vi "HW1.vi"() -> ()   [LabVIEW 2011]
panel:
  out "positive number":dbl
  out "RUNS":i32
  out "RANDOM VALUE CHART":dbl(graph)
  out "RANDOM VALUES\n         (-1 TO 1)":dbl
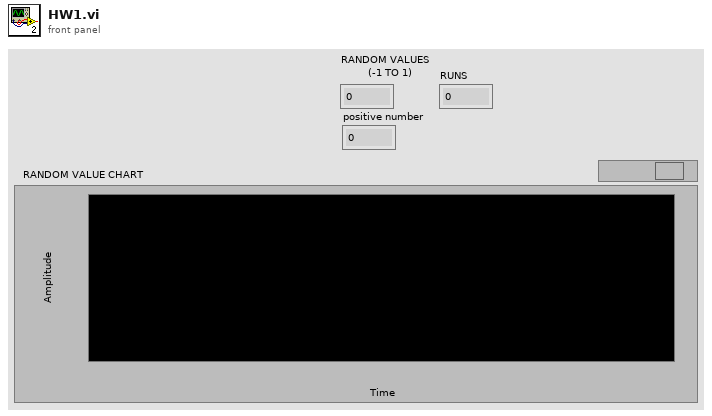
[diagram p1: front panel]
types:
  T1 = enum16{"open", "replace", "create", "open or create", "replace or create", "replace or create with confirmation"}
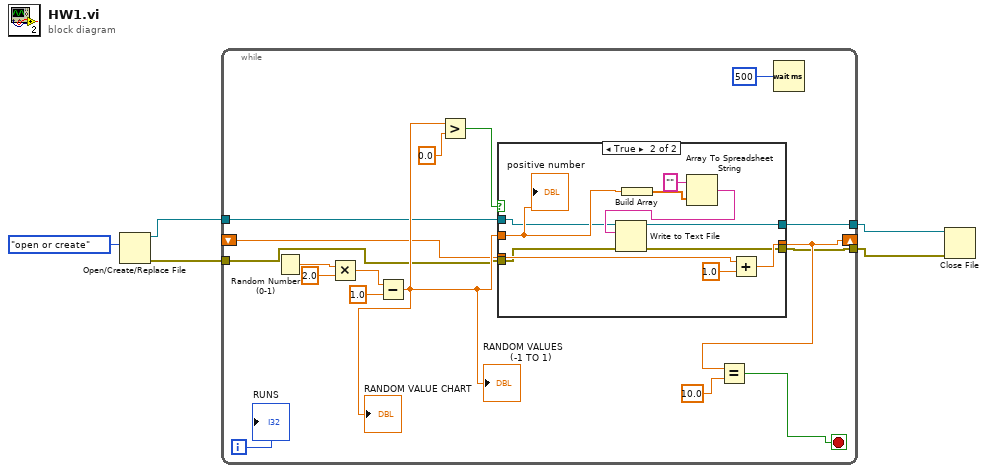
[diagram p0: block diagram]
diagram:
  n1 = Open/Create/Replace File(operation (0:open)=T1."open or create") -> (refnum out=w5:refnum<file>, error out=w3:errorcluster)  [unwired: 5 in, 1 out]
  n2 = while {
    shift-right: [w12] -> _
    shift-left: _ -> [w13]
    tunnel: w5 -> [w9]
    tunnel: [w8] -> w4
    tunnel: w3 -> [w7]
    tunnel: [w6] -> w2
    i -> [w18]
    stop <- w10 stop-if-true
    n3 = Random Number (0-1)() -> (number: 0 to 1=w15:dbl)
    n4 = Multiply(x=w15, y=2.0) -> (x*y=w21:dbl)
    n5 = Subtract(x=w21, y=1.0) -> (x-y=w14:dbl)
    "RANDOM VALUES\n         (-1 TO 1)" <- w14
    "RANDOM VALUE CHART" <- w14
    n6 = Greater?(x=w14, y=0.0) -> (0:w16:bool)
    n7 = case shown="True" w16 {
      tunnel: w14 -> [_ w33]
      tunnel: [w25 w35] -> w12
      tunnel: w13 -> [w25 w34]
      tunnel: w9 -> [w24 w30]
      tunnel: [w24 w29] -> w8
      tunnel: w7 -> [w23 w27]
      tunnel: [w23 w26] -> w6
      frame False {
      }
      frame True {
        n8 = Build Array(w33) -> (w32:dbl[])
        n9 = Array To Spreadsheet String(array=w32, 3:"" ("format string")) -> (spreadsheet string=w31:string)  [unwired: 1 in]
        n10 = Write to Text File(file (use dialog)=w30, text=w31, error in=w27) -> (refnum out=w29:refnum<file>, error out=w26:errorcluster)  [unwired: 1 in, 1 out]
        n11 = Add(x=w34, y=1.0) -> (x+y=w35:dbl)
        "positive number" <- w33
      }
    }
    n12 = Equal?(x=w12, y=10.0) -> (x = y?=w10:bool)
    n13 = Wait (ms)(milliseconds to wait=u32 500) -> ()  [unwired: 1 out]
    "RUNS" <- w18
  }
  n14 = Close File(refnum=w4, error in=w2) -> ()  [unwired: 2 out]
